vi "GetShifterState.vi"(7 "Sensor Failure":bool, 9 "Low Gear Sensor":bool, 10 "High Gear Sensor":bool) -> (2 "Actual Shifter State":T1(ring))   [LabVIEW 2023]
doc: "This VI interpretes the values from two photointerruptor sensors to determine the true current state of the drive module shifting mechanism."
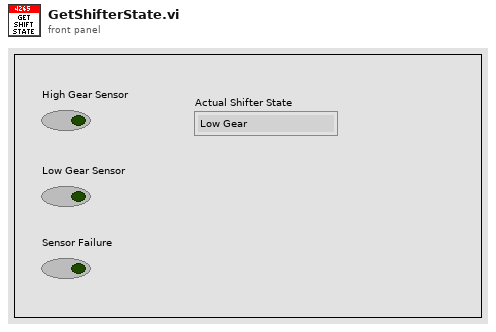
[diagram p1: front panel]
types:
  T1 = enum16{"Low Gear", "High Gear", "Transiting", "Unknown", "Force Low Gear"}
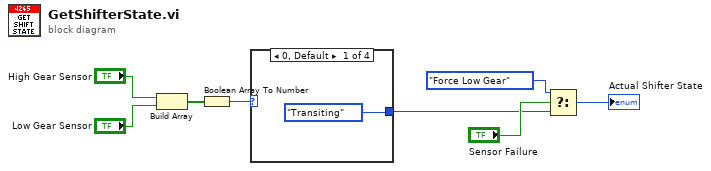
[diagram p0: block diagram]
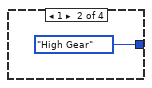
[diagram p2: hidden frame]
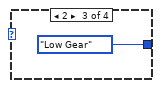
[diagram p3: hidden frame]
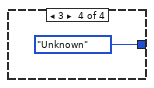
[diagram p4: hidden frame]
diagram:
  n1 = Build Array("High Gear Sensor", "Low Gear Sensor") -> (w6:bool[])
  n2 = Boolean Array To Number(Boolean array=w6) -> (number=w5:u32)
  n3 = case shown="0, Default" w5 {
    tunnel: [T1."Transiting" ("t") T1."High Gear" ("t") T1."Low Gear" ("t") T1."Unknown" ("t")] -> w2
    frame 0, Default {
    }
    frame 1 {
    }
    frame 2 {
    }
    frame 3 {
    }
  }
  n4 = Select(t=T1."Force Low Gear", s="Sensor Failure", f=w2) -> (s? t:f=→"Actual Shifter State":T1)
